vi "Throw Error - Impossible Initial State.vi"(8 "error in":errorcluster, 11 "Explanation":string) -> (0 "error out":errorcluster)   [LabVIEW 2022 SP3]
doc: "Throws a user-generated error that indicates that an impossible initial state was detected."
panel:
  # "Development\ncontrols/indicators useful for development and testing, but which are not outputs of the VI"
  # "Input\nInputs to the VI"
  # "Output\nOutputs of the VI"
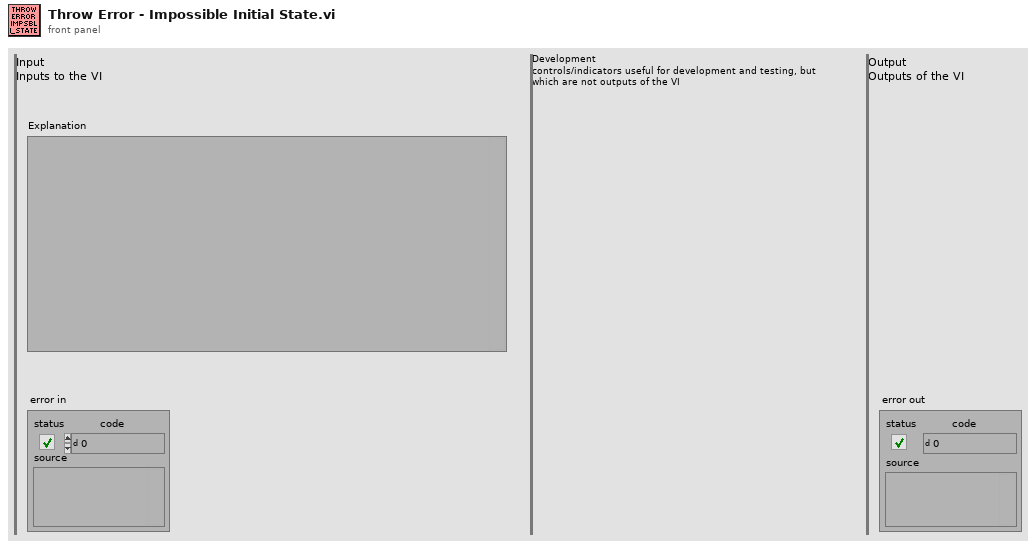
[diagram p1: front panel]
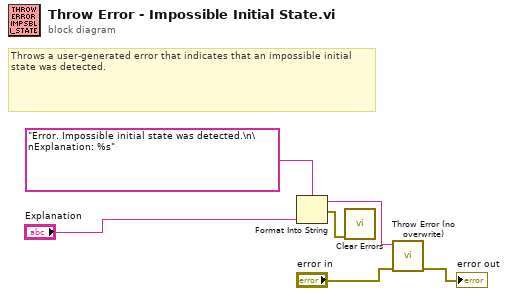
[diagram p0: block diagram]
diagram:
  # "Throws a user-generated error that indicates that an impossible initial state was detected."
  n1 = Format Into String(format string="Error. Impossible initial state was detected.\n\nExplanation: %s", "Explanation") -> (resulting string=w2:string, error out=w1:errorcluster)  [unwired: 2 in]
  n2 = call <vilib>:"Clear Errors.vi"("error in (no error)"=w1) -> ()  [unwired: 5 in, 2 out]
  n3 = call "Throw Error (no overwrite).vi"("error in"="error in", "Error Message"=w2) -> ("error out"=→"error out":errorcluster)  [unwired: 9 in]
